vi "Begin.vi"(8 "error in":errorcluster) -> (0 "error out":errorcluster)   [LabVIEW 2020]
doc: "Called before other user functions, this VI is expected to open initial I/O refnums, load in file data, and do all program initialization. Notice that the <B>error out</B> terminal is simply used for data flow. Wiring it to other structures or subVIs ensures that this VI runs first."
uses:
  <vilib>/Rock Robotics/WPI/DriverStation/WPI_DriverStationRobotMode2.ctl
  <vilib>/Rock Robotics/WPI/Joystick/WPI_JoystickDeviceEnum.ctl
  Robot Global Data.vi
  <vilib>/Rock Robotics/Network Tables/NT Write String Array.vi
  <vilib>/Rock Robotics/WPI/ThirdParty/JAS_Junk/TrajLib/Trajectory_Library.lvlib
  <vilib>/Rock Robotics/SystemInterfaces/spilib/spi_bus.ctl
  <vilib>/Rock Robotics/WPI/Gyro/WPI_GyroXRS450_SPI_Open.vi
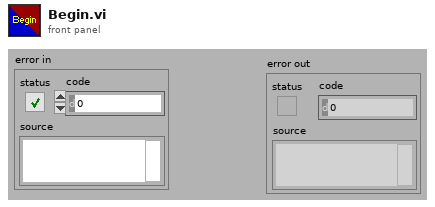
[diagram p1: front panel]
types:
  T1 = typedef "spi_bus.ctl" = enum16{"SPI On-Board, CS0", "SPI On-Board, CS1", "SPI On-Board, CS2", "SPI On-Board, CS3", "SPI MXP", "Invalid"}
  T2 = typedef "WPI_JoystickDeviceEnum.ctl" = enum16{"USB 0", "USB 1", "USB 2", "USB 3", "USB 4", "USB 5"}
  T3 = typedef "WPI_DriverStationRobotMode2.ctl" = enum16{"Autonomous Disabled", "Autonomous Enabled", "Teleop Disabled", "Teleop Enabled", "Disconnected", "Finish", "Test Disabled", "Test Enabled", "Emergency Stopped"}
  T4 = typedef "WPI_JoystickDevRef.ctl" = cluster{"Device":T2}
  T5 = typedef "Trajectory_Library.lvlib/ROTATION2D.ctl" = cluster{"VALUE":dbl, "COS":dbl, "SIN":dbl}
  T6 = typedef "Trajectory_Library.lvlib/SWERVE_DRIVE_MODULE_STATE.ctl" = cluster{"Speed":dbl, "Angle":T5}
  T7 = typedef "Trajectory_Library.lvlib/SWERVE_DRIVE_MODULE_POSITION.ctl" = cluster{"Distance":dbl, "Angle":T5, "P":bool}
  T8 = typedef "Trajectory_Library.lvlib/POSE2D.ctl" = cluster{"TRANSLATION":T9, "ROTATION":T5}
  T9 = typedef "Trajectory_Library.lvlib/TRANSLATION2D.ctl" = cluster{"X":dbl, "Y":dbl}
  T10 = typedef "WPI_MotorControlDeviceRef.ctl" = cluster{"DeviceStatus":errorcluster, "Type":T11, "PWM":cluster{"PWM Channel":T12, "DeadBand":T13}, "CAN":cluster{"Device Number":u8, "SetOutput VI Ref":variant, "GetOutput VI Ref":variant, "Enable VI Ref":variant, "Disable VI Ref":variant, "Data":variant}, "Invert":bool, "DIO PWM":cluster{"PWM \"Enable\" Channel":T12, "DIOChannel":T14, "PWM Rate":dbl}}
  T11 = typedef "WPI_MotorControlType.ctl" = enum16{"PWM", "CAN", "DIO PWM"}
  T12 = typedef "FPGA_DIOPWMChannel.ctl" = enum8{"PWM 0", "PWM 1", "PWM 2", "PWM 3", "PWM 4", "PWM 5", "PWM 6", "PWM 7", "PWM 8", "PWM 9", "PWM MXP 0", "PWM MXP 1", "PWM MXP 2", "PWM MXP 3", "PWM MXP 4", "PWM MXP 5", "PWM MXP 6", "PWM MXP 7", "PWM MXP 8", "PWM MXP 9", "Invalid"}
  T13 = typedef "WPI_PWMDeadband.ctl" = cluster{"Name":string, "maxPositivePwm":i32, "minPositivePwm":i32, "centerPwm":i32, "maxNegativePwm":i32, "minNegativePwm":i32, "angularRange":u16}
  T14 = typedef "FPGA_DIOChannel.ctl" = enum8{"DIO 0", "DIO 1", "DIO 2", "DIO 3", "DIO 4", "DIO 5", "DIO 6", "DIO 7", "DIO 8", "DIO 9", "DIO MXP 0", "DIO MXP 1", "DIO MXP 2", "DIO MXP 3", "DIO MXP 4", "DIO MXP 5", "DIO MXP 6", "DIO MXP 7", "DIO MXP 8", "DIO MXP 9", "DIO MXP 10", "DIO MXP 11", "DIO MXP 12", "DIO MXP 13", "DIO MXP 14", "DIO MXP 15", "SPI Port CS1", "SPI Port CS2", "SPI Port CS3", "SPI Port MISO", "SPI Port MOSI", "Invalid"}
  T15 = typedef "Trajectory_Library.lvlib/SWERVE_DRIVE_ODOMETRY.ctl" = cluster{"POSE":T8, "GyroOffset":T5, "PreviousAngle":T5, "PrevModulePositions":T7[], "NumModules":i32}
  T16 = typedef "WPI_GyroDevRef.ctl" = cluster{"DevStatus":errorcluster, "Analog Channel":T17, "Gain (VoltsPerDegree/Second)":dbl, "Gyro Type":enum16{"Analog", "XRS450"}, "Handle":i32, "SPI Bus":T1, "Device Found":bool, "Sample Rate":dbl, "Calibrate On Open":bool, "Offset":dbl}
  T17 = typedef "FPGA_AIChannel.ctl" = enum8{"AI 0", "AI 1", "AI 2", "AI 3", "AI MXP 0", "AI MXP 1", "AI MXP 2", "AI MXP 3", "Invalid"}
  T18 = cluster{"Max Input ":dbl, "Min Input ":dbl, "Continuous":bool, "Maximum Output":dbl, "Minimum Output ":dbl, "Kn":dbl, "KF":dbl, "KP":dbl, "KI":dbl, "KD":dbl, "Filter Derivative ":bool, "Max Integral":dbl, "Min Integral ":dbl}[]
  T19 = cluster{"Max Input ":dbl, "Min Input ":dbl, "Continuous":bool, "Maximum Output":dbl, "Minimum Output ":dbl, "Kn":dbl, "KF":dbl, "KP":dbl, "KI":dbl, "KD":dbl, "Filter Derivative ":bool, "Max Integral":dbl, "Min Integral ":dbl}
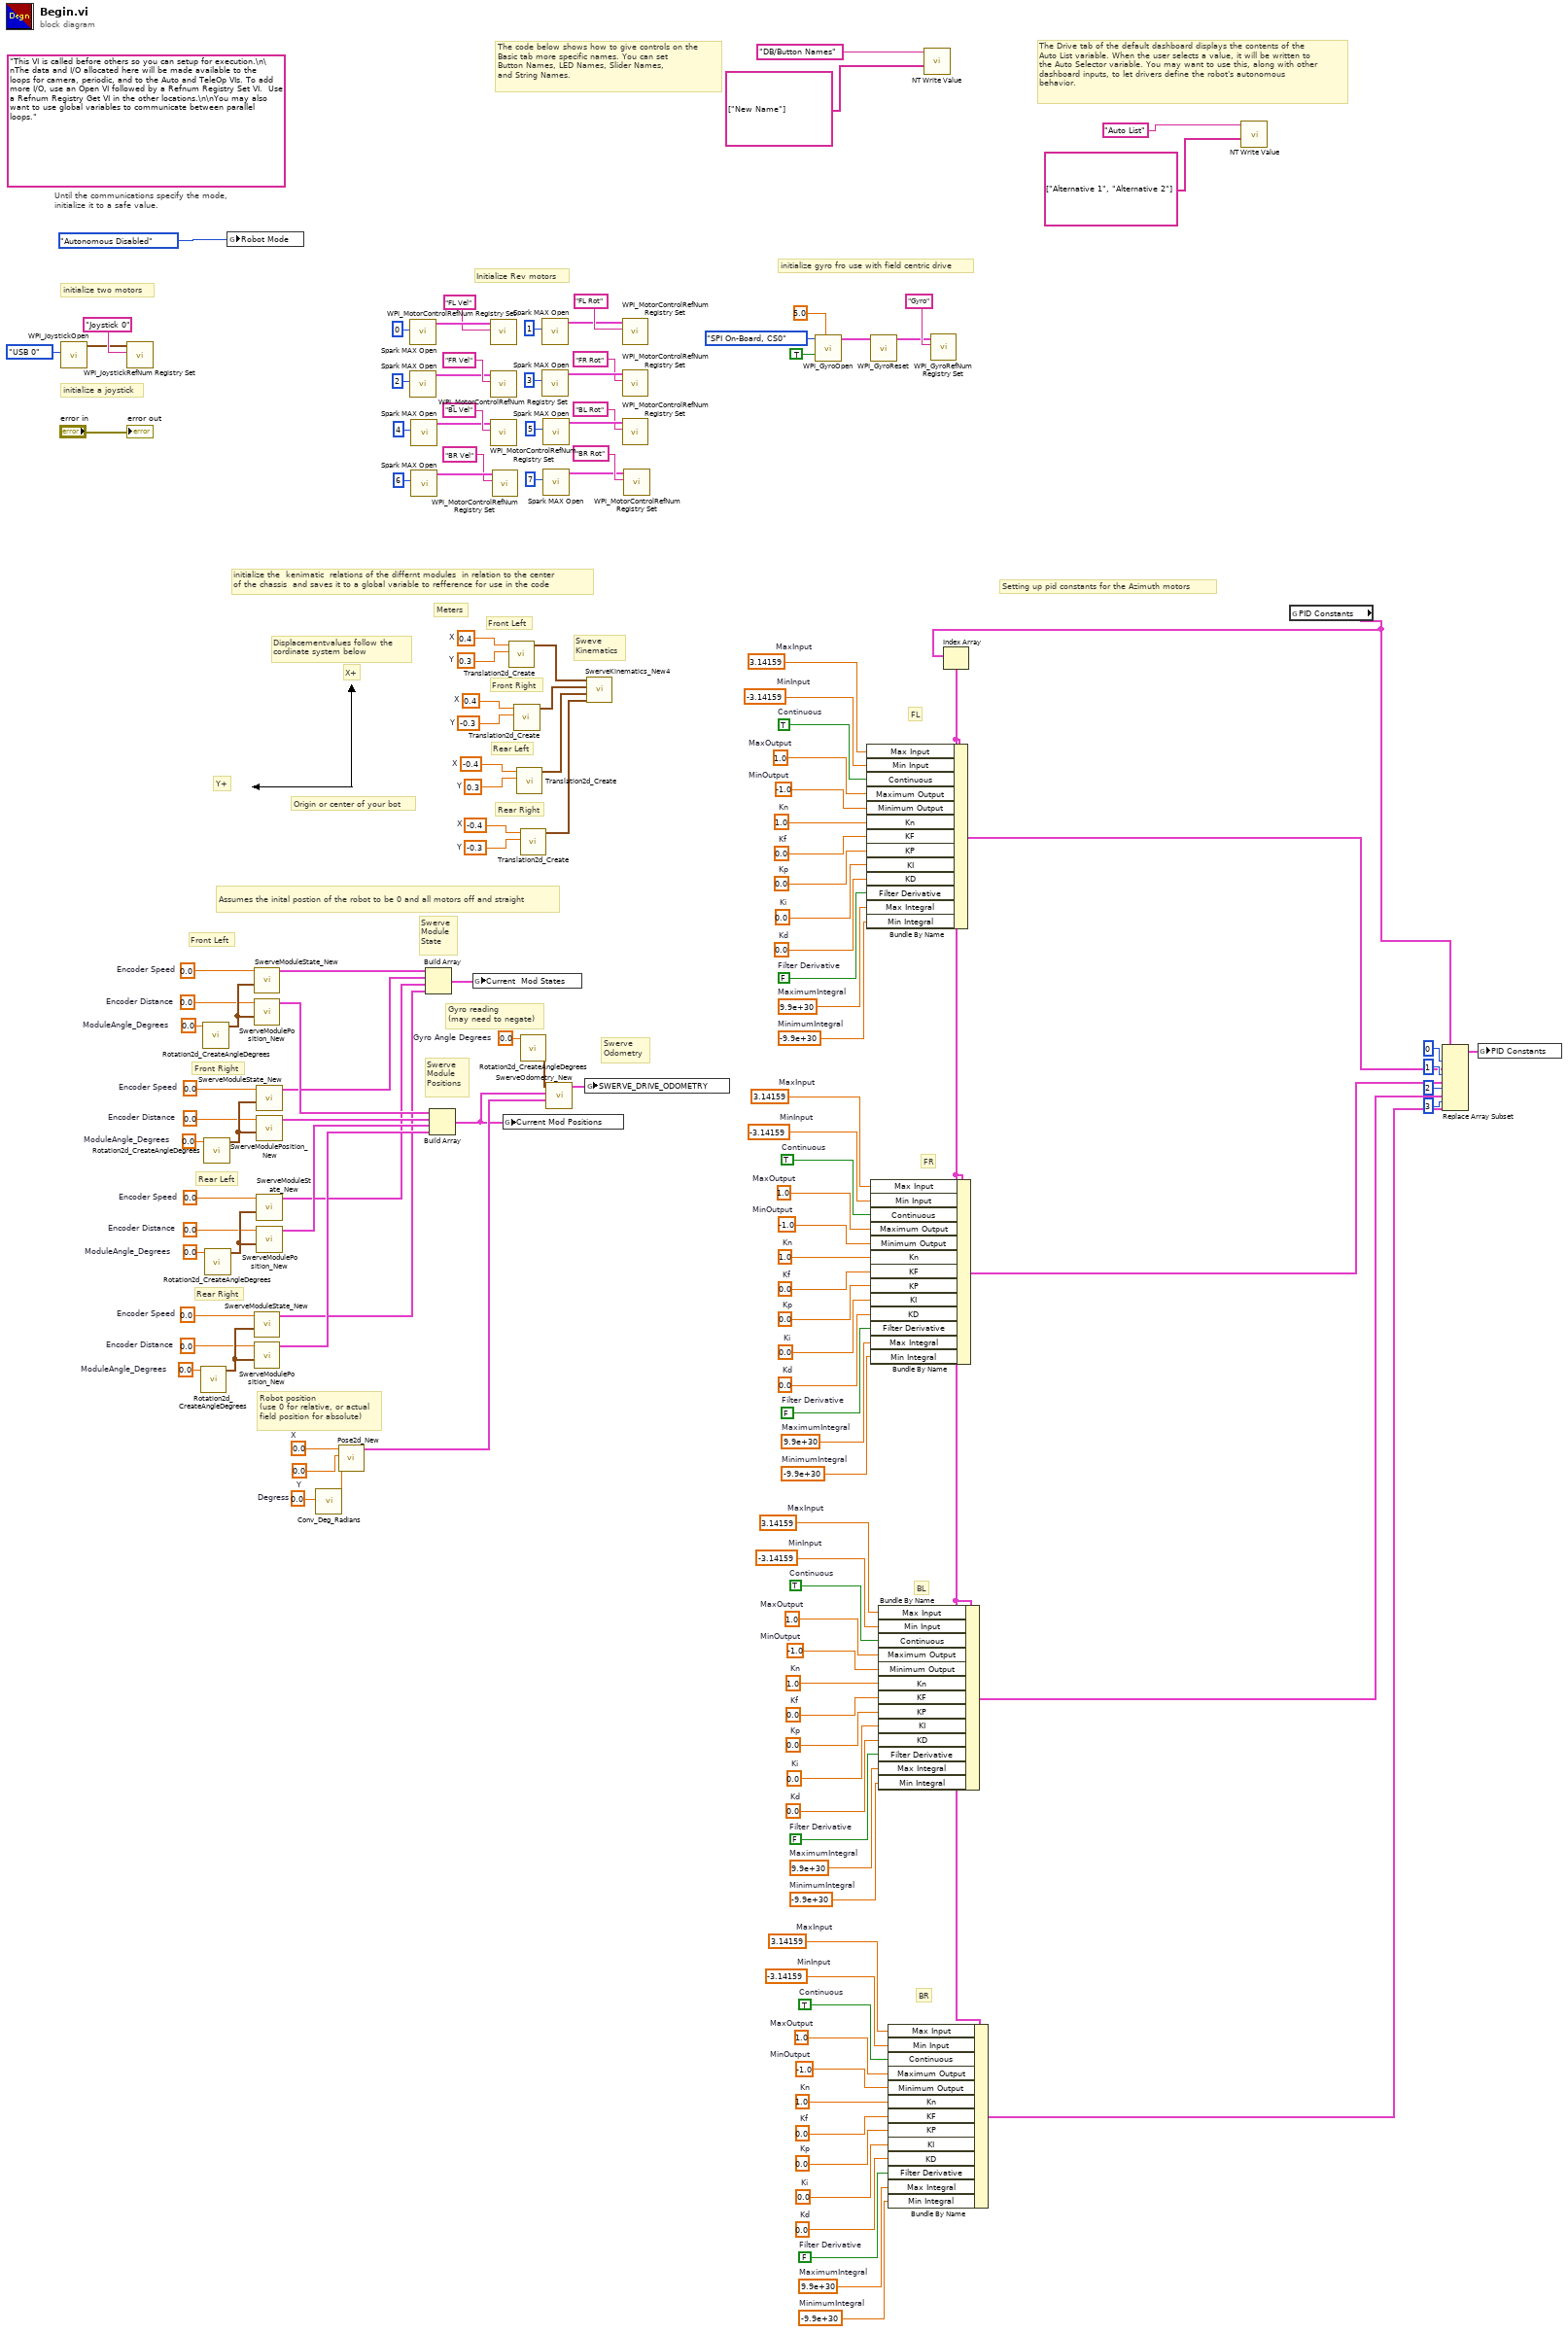
[diagram p0: block diagram]
diagram:
  w20 = 0.0  # Encoder Distance
  w19 = 0.0  # Encoder Distance
  w18 = 0.0  # Encoder Distance
  w16 = 0.0  # Encoder Distance
  w12 = 0.0  # ModuleAngle_Degrees
  w11 = 0.0  # Encoder Speed
  w10 = 0.0  # ModuleAngle_Degrees
  w9 = 0.0  # Encoder Speed
  w8 = 0.0  # ModuleAngle_Degrees
  w7 = 0.0  # Encoder Speed
  w5 = 0.0  # ModuleAngle_Degrees
  w4 = 0.0  # Encoder Speed
  w33 = 0.0  # Degress
  w32 = 0.0  # X
  w31 = 0.0  # Y
  w28 = 0.0  # Gyro Angle Degrees
  w45 = 1.0  # Kn
  w47 = 0.0  # Kp
  w48 = 0.0  # Ki
  w49 = 0.0  # Kd
  w46 = 0.0  # Kf
  w50 = 9.9e+30  # MaximumIntegral
  w51 = -9.9e+30  # MinimumIntegral
  w52 = FALSE  # Filter Derivative
  w41 = -3.14159  # MinInput
  w42 = TRUE  # Continuous
  w43 = 1.0  # MaxOutput
  w44 = -1.0  # MinOutput
  w40 = 3.14159  # MaxInput
  w60 = 1.0  # Kn
  w58 = 0.0  # Kp
  w57 = 0.0  # Ki
  w56 = 0.0  # Kd
  w59 = 0.0  # Kf
  w55 = 9.9e+30  # MaximumIntegral
  w54 = -9.9e+30  # MinimumIntegral
  w53 = FALSE  # Filter Derivative
  w64 = -3.14159  # MinInput
  w63 = TRUE  # Continuous
  w62 = 1.0  # MaxOutput
  w61 = -1.0  # MinOutput
  w65 = 3.14159  # MaxInput
  w71 = 1.0  # Kn
  w73 = 0.0  # Kp
  w74 = 0.0  # Ki
  w75 = 0.0  # Kd
  w72 = 0.0  # Kf
  w76 = 9.9e+30  # MaximumIntegral
  w77 = -9.9e+30  # MinimumIntegral
  w78 = FALSE  # Filter Derivative
  w67 = -3.14159  # MinInput
  w68 = TRUE  # Continuous
  w69 = 1.0  # MaxOutput
  w70 = -1.0  # MinOutput
  w66 = 3.14159  # MaxInput
  w86 = 1.0  # Kn
  w84 = 0.0  # Kp
  w83 = 0.0  # Ki
  w82 = 0.0  # Kd
  w85 = 0.0  # Kf
  w81 = 9.9e+30  # MaximumIntegral
  w80 = -9.9e+30  # MinimumIntegral
  w79 = FALSE  # Filter Derivative
  w90 = -3.14159  # MinInput
  w89 = TRUE  # Continuous
  w88 = 1.0  # MaxOutput
  w87 = -1.0  # MinOutput
  w91 = 3.14159  # MaxInput
  w111 = -0.4  # X
  w110 = -0.3  # Y
  w109 = -0.4  # X
  w108 = 0.3  # Y
  w107 = 0.4  # X
  w106 = -0.3  # Y
  w105 = 0.4  # X
  w104 = 0.3  # Y
  (unwired) "This VI is called before others so you can setup for execution.\n\nThe data and I/O allocated here will be made available to the loops for camera, periodic, and to the Auto and TeleOp VIs. To add more I/O, use an Open VI followed by a Refnum Registry Set VI.  Use a Refnum Registry Get VI in the other locations.\n\nYou may also want to use global variables to communicate between parallel loops."
  # "Assumes the inital postion of the robot to be 0 and all motors off and straight"
  # "Swerve\nModule\nPositions"
  # "Front Left"
  # "Swerve\nModule\nState"
  # "Rear Right"
  # "Rear Left"
  # "Front Right"
  # "Swerve\nOdometry"
  # "Robot position\n(use 0 for relative, or actual \nfield position for absolute)"
  # "Gyro reading\n(may need to negate)"
  # "BR"
  # "BL"
  # "FR"
  # "FL"
  # "Setting up pid constants for the Azimuth motors"
  # "initialize gyro fro use with field centric drive"
  # "Origin or center of your bot"
  # "Y+"
  # "X+"
  # "Displacementvalues follow the \ncordinate system below"
  # "initialize the  kenimatic  relations of the differnt modules  in relation to the center \nof the chassis  and saves it to a global variable to refference for use in the code"
  # "Meters"
  # "Sweve\nKinematics"
  # "Rear Right"
  # "Rear Left"
  # "Front Right"
  # "Front Left"
  # "Initialize Rev motors"
  # "The Drive tab of the default dashboard displays the contents of the\nAuto List variable. When the user selects a value, it will be written to\nthe Auto Selector variable. You may want to use this, along with other\ndashboard inputs, to let drivers define the robot's autonomous\nbehavior."
  # "The code below shows how to give controls on the\nBasic tab more specific names. You can set\nButton Names, LED Names, Slider Names,\nand String Names."
  # "initialize a joystick"
  # "Until the communications specify the mode,\ninitialize it to a safe value."
  # "initialize two motors"
  n1 = call <vilib>:"WPI_JoystickOpen.vi"("JoystickDevice"=WPI_JoystickDeviceEnum."USB 0") -> ("JoystickDevRef"=w146:T4)  [unwired: 10 in]
  n2 = call <vilib>:"WPI_JoystickRefNum Registry Set.vi"("refnum name"="Joystick 0", "JoystickDevRef"=w146) -> ()  [unwired: 8 in, 2 out]
  n3 = call <vilib>:"Rotation2d_CreateAngleDegrees.vi"("Angle_Degrees"=w12) -> ("ROTATION"=w27:T5)  [unwired: 10 in]
  n4 = call <vilib>:"Rotation2d_CreateAngleDegrees.vi"("Angle_Degrees"=w5) -> ("ROTATION"=w24:T5)  [unwired: 10 in]
  n5 = call <vilib>:"Rotation2d_CreateAngleDegrees.vi"("Angle_Degrees"=w8) -> ("ROTATION"=w25:T5)  [unwired: 10 in]
  n6 = call <vilib>:"Rotation2d_CreateAngleDegrees.vi"("Angle_Degrees"=w10) -> ("ROTATION"=w26:T5)  [unwired: 10 in]
  n7 = global write "Robot Global Data.vi" "Robot Mode"(WPI_DriverStationRobotMode2."Autonomous Disabled" ("Robot Mode")) -> ()
  n8 = call <vilib>:"SwerveModuleState_New.vi"("ROTATION"=w24, "Speed"=w4) -> ("SWERVE_DRIVE_MODULE_STATE"=w6:T6)  [unwired: 9 in]
  n9 = call <vilib>:"SwerveModulePosition_New.vi"("ROTATION"=w24, "Distance"=w16) -> ("SWERVE_DRIVE_MODULE_POSITION"=w17:T7)  [unwired: 9 in]
  n10 = call <vilib>:"SwerveModuleState_New.vi"("ROTATION"=w27, "Speed"=w11) -> ("SWERVE_DRIVE_MODULE_STATE"=w15:T6)  [unwired: 9 in]
  n11 = call <vilib>:"SwerveModulePosition_New.vi"("ROTATION"=w27, "Distance"=w20) -> ("SWERVE_DRIVE_MODULE_POSITION"=w23:T7)  [unwired: 9 in]
  n12 = call <vilib>:"SwerveModuleState_New.vi"("ROTATION"=w25, "Speed"=w7) -> ("SWERVE_DRIVE_MODULE_STATE"=w13:T6)  [unwired: 9 in]
  n13 = call <vilib>:"SwerveModulePosition_New.vi"("ROTATION"=w25, "Distance"=w18) -> ("SWERVE_DRIVE_MODULE_POSITION"=w21:T7)  [unwired: 9 in]
  n14 = call <vilib>:"SwerveModuleState_New.vi"("ROTATION"=w26, "Speed"=w9) -> ("SWERVE_DRIVE_MODULE_STATE"=w14:T6)  [unwired: 9 in]
  n15 = call <vilib>:"SwerveModulePosition_New.vi"("ROTATION"=w26, "Distance"=w19) -> ("SWERVE_DRIVE_MODULE_POSITION"=w22:T7)  [unwired: 9 in]
  n16 = call <vilib>:"Conv_Deg_Radians.vi"("Degress"=w33) -> ("Radians"=w30:dbl)  [unwired: 10 in]
  n17 = call <vilib>:"Pose2d_New.vi"("Heading"=w30, "Y"=w31, "X"=w32) -> ("out POSe"=w34:T8)  [unwired: 8 in]
  n18 = call <vilib>:"Spark MAX Open.vi"("Device Number"=u8 0) -> ("MotorControlDeviceRef"=w139:T10)  [unwired: 9 in, 1 out]
  n19 = call <vilib>:"Spark MAX Open.vi"("Device Number"=u8 2) -> ("MotorControlDeviceRef"=w136:T10)  [unwired: 9 in, 1 out]
  n20 = call <vilib>:"Spark MAX Open.vi"("Device Number"=u8 4) -> ("MotorControlDeviceRef"=w132:T10)  [unwired: 9 in, 1 out]
  n21 = call <vilib>:"Spark MAX Open.vi"("Device Number"=u8 6) -> ("MotorControlDeviceRef"=w135:T10)  [unwired: 9 in, 1 out]
  n22 = Build Array(w6, w13, w14, w15) -> (w3:T6[])
  n23 = Build Array(w17, w21, w22, w23) -> (w2:T7[])
  n24 = global write "Robot Global Data.vi" "Current  Mod States"(w3) -> ()
  n25 = call <vilib>:"WPI_MotorControlRefNum Registry Set.vi"("refnum name"="FL Vel", "MotorControlDevRef"=w139) -> ()  [unwired: 8 in, 2 out]
  n26 = call <vilib>:"WPI_MotorControlRefNum Registry Set.vi"("refnum name"="FR Vel", "MotorControlDevRef"=w136) -> ()  [unwired: 8 in, 2 out]
  n27 = call <vilib>:"WPI_MotorControlRefNum Registry Set.vi"("refnum name"="BL Vel", "MotorControlDevRef"=w132) -> ()  [unwired: 8 in, 2 out]
  n28 = call <vilib>:"WPI_MotorControlRefNum Registry Set.vi"("refnum name"="BR Vel", "MotorControlDevRef"=w135) -> ()  [unwired: 8 in, 2 out]
  n29 = global write "Robot Global Data.vi" "Current Mod Positions"(w2) -> ()
  n30 = call <vilib>:"Translation2d_Create.vi"("Y"=w104, "X"=w105) -> ("TRANSLATION"=w112:T9)  [unwired: 9 in]
  n31 = call <vilib>:"Translation2d_Create.vi"("Y"=w106, "X"=w107) -> ("TRANSLATION"=w113:T9)  [unwired: 9 in]
  n32 = call <vilib>:"Translation2d_Create.vi"("Y"=w108, "X"=w109) -> ("TRANSLATION"=w114:T9)  [unwired: 9 in]
  n33 = call <vilib>:"Translation2d_Create.vi"("Y"=w110, "X"=w111) -> ("TRANSLATION"=w115:T9)  [unwired: 9 in]
  n34 = call <vilib>:"Rotation2d_CreateAngleDegrees.vi"("Angle_Degrees"=w28) -> ("ROTATION"=w29:T5)  [unwired: 10 in]
  n35 = call <vilib>:"Spark MAX Open.vi"("Device Number"=u8 1) -> ("MotorControlDeviceRef"=w124:T10)  [unwired: 9 in, 1 out]
  n36 = call <vilib>:"Spark MAX Open.vi"("Device Number"=u8 3) -> ("MotorControlDeviceRef"=w127:T10)  [unwired: 9 in, 1 out]
  n37 = call <vilib>:"Spark MAX Open.vi"("Device Number"=u8 5) -> ("MotorControlDeviceRef"=w131:T10)  [unwired: 9 in, 1 out]
  n38 = call <vilib>:"Spark MAX Open.vi"("Device Number"=u8 7) -> ("MotorControlDeviceRef"=w128:T10)  [unwired: 9 in, 1 out]
  n39 = call <vilib>:"SwerveOdometry_New.vi"("InitialPose"=w34, "Module Positions"=w2, "gyroAngle"=w29) -> ("SWERVE_DRIVE_ODOMETRY"=w1:T15)  [unwired: 8 in]
  n40 = global write "Robot Global Data.vi" "SWERVE_DRIVE_ODOMETRY"(w1) -> ()
  n41 = call <vilib>:"SwerveKinematics_New4.vi"("wheel 3"=w115, "wheel 2"=w114, "wheel 1"=w113, "wheel 0"=w112) -> ()  [unwired: 7 in, 1 out]
  n42 = call <vilib>:"WPI_MotorControlRefNum Registry Set.vi"("refnum name"="FL Rot", "MotorControlDevRef"=w124) -> ()  [unwired: 8 in, 2 out]
  n43 = call <vilib>:"WPI_MotorControlRefNum Registry Set.vi"("refnum name"="FR Rot", "MotorControlDevRef"=w127) -> ()  [unwired: 8 in, 2 out]
  n44 = call <vilib>:"WPI_MotorControlRefNum Registry Set.vi"("refnum name"="BL Rot", "MotorControlDevRef"=w131) -> ()  [unwired: 8 in, 2 out]
  n45 = call <vilib>:"WPI_MotorControlRefNum Registry Set.vi"("refnum name"="BR Rot", "MotorControlDevRef"=w128) -> ()  [unwired: 8 in, 2 out]
  n46 = call-poly <vilib>:"WPI_GyroOpen.vi"("Calibration Time (s)"=5.0, "Calibrate On Open"=TRUE, "SPI Bus"=spi_bus."SPI On-Board, CS0") -> ("GyroDevRef"=w101:T16)  [unwired: 6 in, 2 out]
  n47 = call <vilib>:"WPI_GyroReset.vi"("GyroDevRef"=w101) -> ("GyroDevRef"=w102:T16)  [unwired: 9 in, 1 out]
  n48 = call-poly <vilib>:"NT Write Value.vi"("value"=string[] ["New Name"], "name"="DB/Button Names" ("Name")) -> ()  [unwired: 9 in, 1 out]
  n49 = call <vilib>:"WPI_GyroRefNum Registry Set.vi"("refnum name"="Gyro", "GyroDevRef"=w102) -> ()  [unwired: 8 in, 2 out]
  n50 = call-poly <vilib>:"NT Write Value.vi"("value"=string[] ["Alternative 1", "Alternative 2"] ("String Array"), "name"="Auto List" ("Name")) -> ()  [unwired: 9 in, 1 out]
  n51 = global read "Robot Global Data.vi" "PID Constants"() -> (w97:T18)
  n52 = Index Array(array=w97) -> (element=w39:T19)  [unwired: 1 in]
  n53 = Bundle By Name(cluster=w39, "Max Input"=w91, "Min Input"=w90, "Continuous"=w89, "Maximum Output"=w88, "Minimum Output"=w87, "Kn"=w86, "KF"=w85, "KP"=w84, "KI"=w83, "KD"=w82, "Filter Derivative"=w79, "Max Integral"=w81, "Min Integral"=w80) -> (w92:T19)
  n54 = Bundle By Name(cluster=w39, "Max Input"=w66, "Min Input"=w67, "Continuous"=w68, "Maximum Output"=w69, "Minimum Output"=w70, "Kn"=w71, "KF"=w72, "KP"=w73, "KI"=w74, "KD"=w75, "Filter Derivative"=w78, "Max Integral"=w76, "Min Integral"=w77) -> (w38:T19)
  n55 = Bundle By Name(cluster=w39, "Max Input"=w65, "Min Input"=w64, "Continuous"=w63, "Maximum Output"=w62, "Minimum Output"=w61, "Kn"=w60, "KF"=w59, "KP"=w58, "KI"=w57, "KD"=w56, "Filter Derivative"=w53, "Max Integral"=w55, "Min Integral"=w54) -> (w37:T19)
  n56 = Bundle By Name(cluster=w39, "Max Input"=w40, "Min Input"=w41, "Continuous"=w42, "Maximum Output"=w43, "Minimum Output"=w44, "Kn"=w45, "KF"=w46, "KP"=w47, "KI"=w48, "KD"=w49, "Filter Derivative"=w52, "Max Integral"=w50, "Min Integral"=w51) -> (w36:T19)
  n57 = Replace Array Subset(array=w97, new element #1=w92, index #1=0 ("index"), new element #2=w38, index #2=1 ("index"), new element #3=w37, index #3=2 ("index"), new element #4=w36, index #4=3 ("index")) -> (w35:T18)
  n58 = global write "Robot Global Data.vi" "PID Constants"(w35) -> ()
  "error out" <- "error in"
